vi "returnState.vi"(6 "error IN":errorcluster, 8 "String IN":string) -> (0 "error out":errorcluster, 1 "Return State":T2(ring), 3 "output cluster":T1)   [LabVIEW 2017]
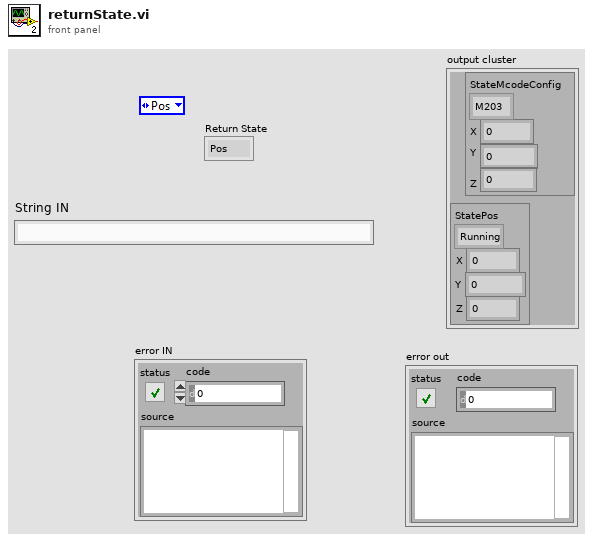
[diagram p1: front panel]
types:
  T1 = cluster{"OUTCONFIG":cluster{"StateMcodeConfig":enum16{"M203", "M201", "M92", "M3001"}, "X":dbl, "Y":dbl, "Z":dbl}, "outPOS":cluster{"StatePos":enum16{"Running", "Waiting", "Pos", "IDLE"}, "X":dbl, "Z":dbl, "Y":dbl}}
  T2 = enum16{"Pos", "Config", "Data1", "Data2", "Step", "Error"}
  T3 = enum16{"Pos", "Config", "Data1", "Data2", "Step"}
  T4 = cluster{"Enum":enum16{"Running", "Waiting", "Pos", "IDLE"}, dbl, dbl, dbl}
  T5 = cluster{"StateMcodeConfig":enum16{"M203", "M201", "M92", "M3001"}, dbl, dbl, dbl}
  T6 = cluster{cluster{"StateMcodeConfig":enum16{"M203", "M201", "M92", "M3001"}, dbl, dbl, dbl}, cluster{"Enum":enum16{"Running", "Waiting", "Pos", "IDLE"}, dbl, dbl, dbl}}
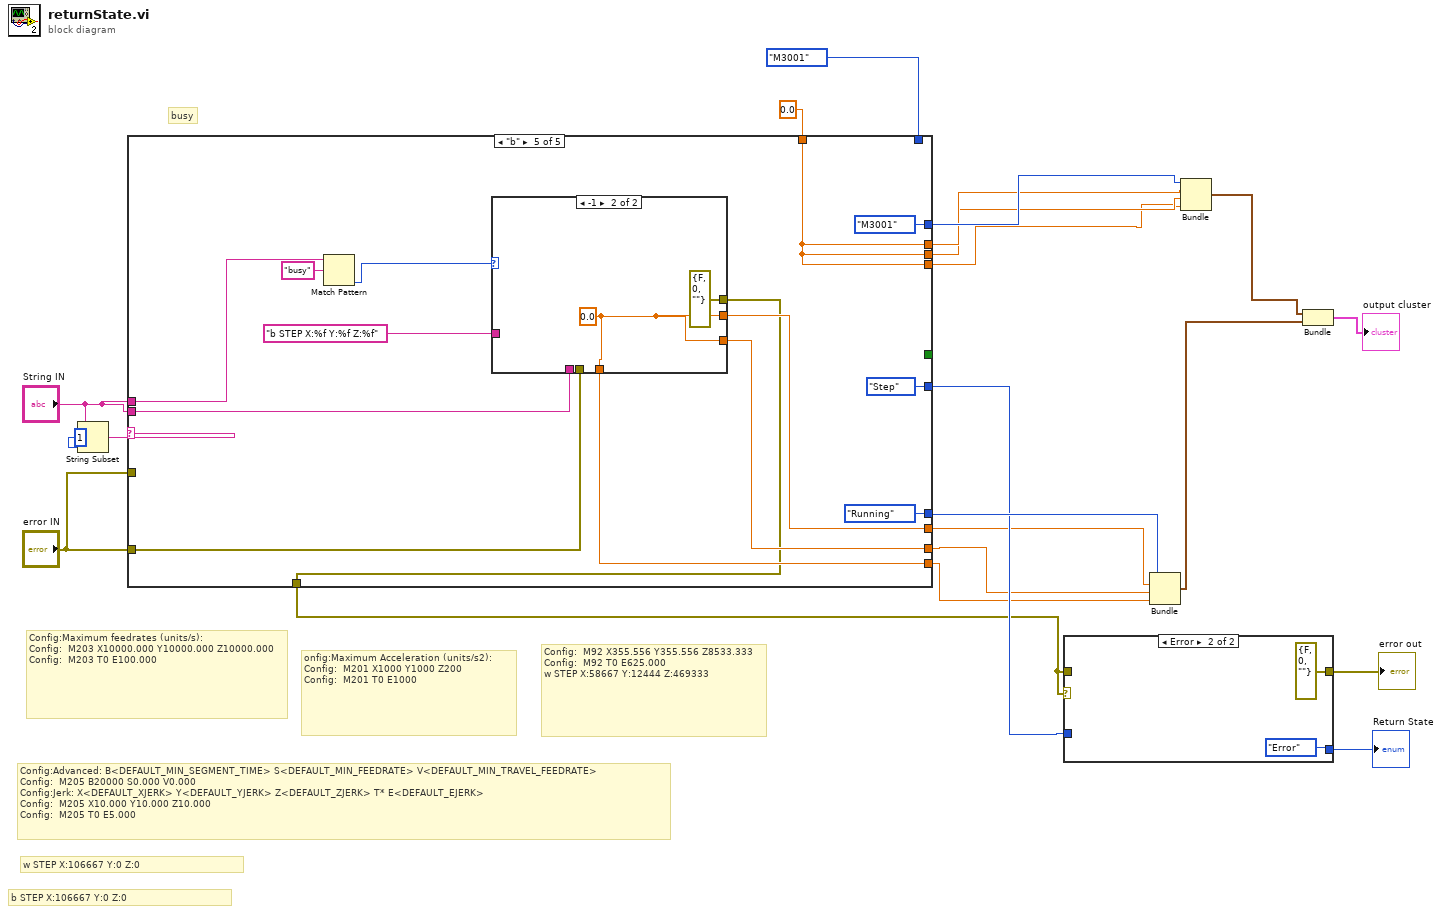
[diagram p0: block diagram]
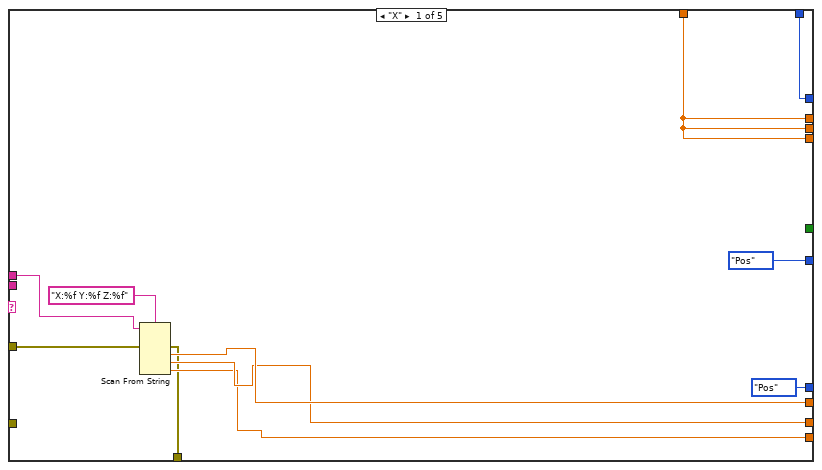
[diagram p3: hidden frame]
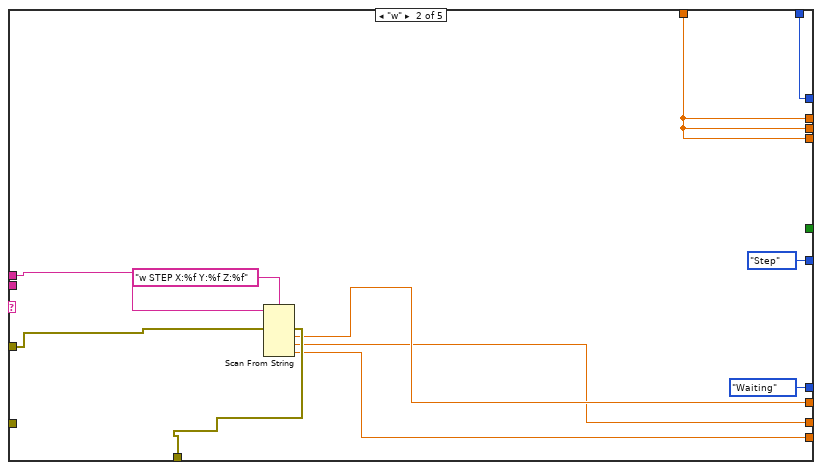
[diagram p4: hidden frame]
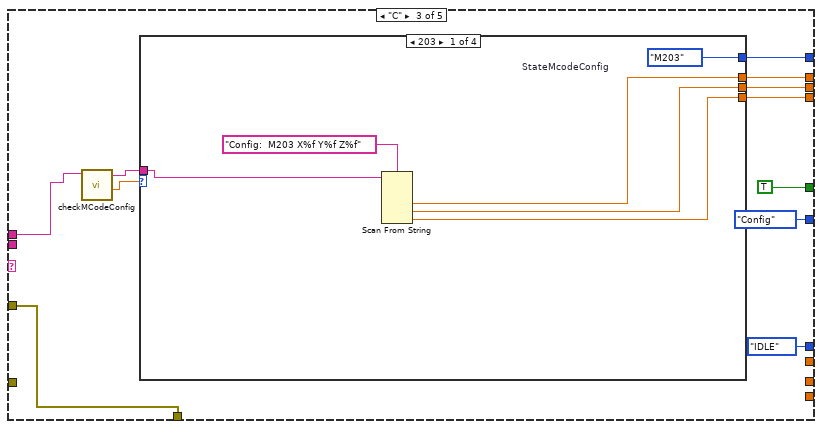
[diagram p5: hidden frame]
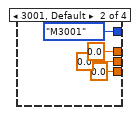
[diagram p6: hidden frame]
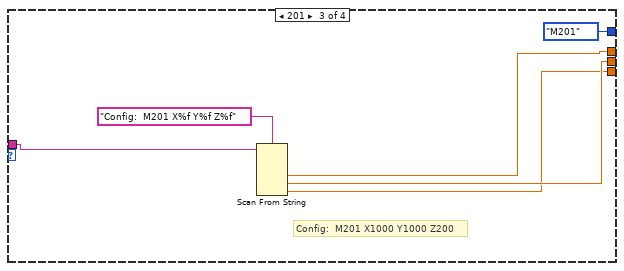
[diagram p7: hidden frame]
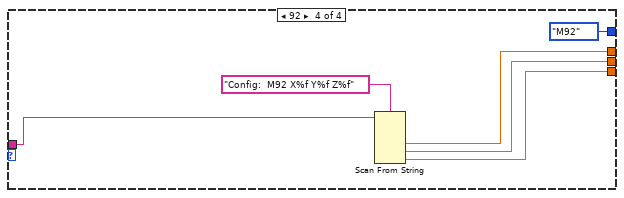
[diagram p8: hidden frame]
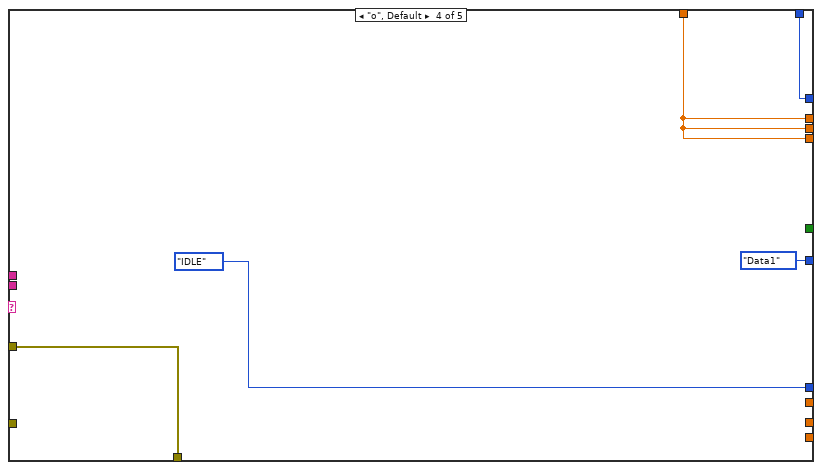
[diagram p9: hidden frame]
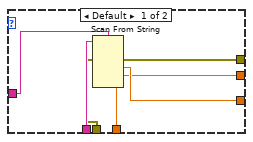
[diagram p10: hidden frame]
diagram:
  # "busy"
  # "b STEP X:106667 Y:0 Z:0"
  # "Config:Advanced: B<DEFAULT_MIN_SEGMENT_TIME> S<DEFAULT_MIN_FEEDRATE> V<DEFAULT_MIN_TRAVEL_FEEDRATE>\nConfig:  M205 B20000 S0.000 V0.000\nConfig:Jerk: X<DEFAULT_XJERK> Y<DEFAULT_YJERK> Z<DEFAULT_ZJERK> T* E<DEFAULT_EJERK>\nConfig:  M205 X10.000 Y10.000 Z10.000\nConfig:  M205 T0 E5.000"
  # "Config:  M92 X355.556 Y355.556 Z8533.333\nConfig:  M92 T0 E625.000\nw STEP X:58667 Y:12444 Z:469333"
  # "onfig:Maximum Acceleration (units/s2):\nConfig:  M201 X1000 Y1000 Z200\nConfig:  M201 T0 E1000"
  # "Config:Maximum feedrates (units/s):\nConfig:  M203 X10000.000 Y10000.000 Z10000.000\nConfig:  M203 T0 E100.000"
  # "w STEP X:106667 Y:0 Z:0"
  n1 = String Subset(string="String IN", length (rest)=1 ("length (rest)")) -> (substring=w20:string)  [unwired: 1 in]
  n2 = case shown="\"b\"" w20 {
    tunnel: [enum16{"Running", "Waiting", "Pos", "IDLE"}."Pos" ("Enum") enum16{"Running", "Waiting", "Pos", "IDLE"}."Waiting" ("Enum") enum16{"Running", "Waiting", "Pos", "IDLE"}."IDLE" ("Enum") enum16{"Running", "Waiting", "Pos", "IDLE"}."IDLE" ("Enum") enum16{"Running", "Waiting", "Pos", "IDLE"}."Running" ("Enum")] -> w19
    tunnel: "String IN" -> [w31 w42 w52 _ w91]
    tunnel: [w30 w39 _ _ w83] -> w3
    tunnel: [w29 w38 _ _ w84] -> w2
    tunnel: [w28 w35 _ _ w85] -> w4
    tunnel: "error IN" -> [w27 w41 w54 w80 _]
    tunnel: [w26 w40 w54 w80 w82] -> w1
    tunnel: [w25 w36 w49 w78 w94] -> w15
    tunnel: [w25 w36 w48 w78 w94] -> w14
    tunnel: [w25 w36 w47 w78 w94] -> w13
    tunnel: [w23 w37 w46 w79 enum16{"M203", "M201", "M92", "M3001"}."M3001" ("StateMcodeConfig")] -> w16
    tunnel: enum16{"M203", "M201", "M92", "M3001"}."M3001" ("StateMcodeConfig") -> [w23 w37 _ w79 _]
    tunnel: 0.0 -> [w25 w36 _ w78 w94]
    tunnel: [_ _ TRUE ("Status") _ _] -> _
    tunnel: [T3."Pos" ("Return State") T3."Step" ("Return State") T3."Config" ("Return State") T3."Data1" ("Return State") T2."Step" ("Return State")] -> w8
    tunnel: "String IN" -> [_ _ _ _ w87]
    tunnel: "error IN" -> [_ _ _ _ w86]
    frame "X" {
      n3 = Scan From String(format string="X:%f Y:%f Z:%f", input string=w31, error in=w27) -> (error out=w26:errorcluster, output 1=w30:dbl, output 2=w29:dbl, output 3=w28:dbl)  [unwired: 4 in, 2 out]
    }
    frame "w" {
      n4 = Scan From String(format string="w STEP X:%f Y:%f Z:%f", input string=w42, error in=w41) -> (error out=w40:errorcluster, output 1=w39:dbl, output 2=w38:dbl, output 3=w35:dbl)  [unwired: 4 in, 2 out]
    }
    frame "C" {
      n5 = call "checkMCodeConfig.vi"("INPUT"=w52) -> ("MCODE"=w51:dbl, "OUTPUT"=w50:string)  [unwired: 9 in]
      n6 = case shown="203" w51 {
        tunnel: w50 -> [w59 _ w69 w75]
        tunnel: [w58 0.0 w68 w74] -> w49
        tunnel: [w57 0.0 w67 w73] -> w48
        tunnel: [w56 0.0 w66 w72] -> w47
        tunnel: [w55 enum16{"M203", "M201", "M92", "M3001"}."M3001" ("StateMcodeConfig") enum16{"M203", "M201", "M92", "M3001"}."M201" ("StateMcodeConfig") enum16{"M203", "M201", "M92", "M3001"}."M92" ("StateMcodeConfig")] -> w46
        frame 203 {
          w55 = enum16{"M203", "M201", "M92", "M3001"}."M203"  # StateMcodeConfig
          n7 = Scan From String(format string="Config:  M203 X%f Y%f Z%f", input string=w59) -> (output 1=w58:dbl, output 2=w57:dbl, output 3=w56:dbl)  [unwired: 5 in, 3 out]
        }
        frame 3001, Default {
        }
        frame 201 {
          # "Config:  M201 X1000 Y1000 Z200"
          n8 = Scan From String(format string="Config:  M201 X%f Y%f Z%f", input string=w69) -> (output 1=w68:dbl, output 2=w67:dbl, output 3=w66:dbl)  [unwired: 5 in, 3 out]
        }
        frame 92 {
          n9 = Scan From String(format string="Config:  M92 X%f Y%f Z%f", input string=w75) -> (output 1=w74:dbl, output 2=w73:dbl, output 3=w72:dbl)  [unwired: 5 in, 3 out]
        }
      }
    }
    frame "o", Default {
    }
    frame "b" {
      n10 = Match Pattern(string=w91, regular expression="busy") -> (offset past match=w89:i32)  [unwired: 1 in, 3 out]
      n11 = case shown="-1" w89 {
        tunnel: "b STEP X:%f Y:%f Z:%f" ("format string") -> [w102 _]
        tunnel: w87 -> [w101 _]
        tunnel: w86 -> [w100 _]
        tunnel: [w99 errorcluster {"status"=FALSE, "code"=0, "source"=""} ("error IO")] -> w82
        tunnel: [w98 w103] -> w84
        tunnel: [w97 w103] -> w83
        tunnel: [w96 w103] -> w85
        frame Default {
          n12 = Scan From String(format string=w102, input string=w101, error in=w100) -> (error out=w99:errorcluster, output 1=w98:dbl, output 2=w97:dbl, output 3=w96:dbl)  [unwired: 4 in, 2 out]
        }
        frame -1 {
          w103 = 0.0
        }
      }
    }
  }
  n13 = case shown="Error" w1 {
    tunnel: w1 -> [w106 _]
    tunnel: [w106 errorcluster {"status"=FALSE, "code"=0, "source"=""} ("error IO")] -> w9
    tunnel: w8 -> [w105 _]
    tunnel: [w105 T2."Error" ("Return State")] -> w7
    frame No Error {
    }
    frame Error {
    }
  }
  "error out" <- w9
  "Return State" <- w7
  n14 = Bundle("Enum"=w19, w3, w2, w4) -> (w11:T4)  [unwired: 1 in]
  n15 = Bundle("StateMcodeConfig"=w16, w15, w14, w13) -> (w10:T5)  [unwired: 1 in]
  n16 = Bundle(w10, w11) -> (→"output cluster":T6)  [unwired: 1 in]
